vi "onTestExecution.vi"(7 "Name":string, 8 "error in (no error)":errorcluster, 11 "Test Runner in":refnum<class "Test Runner.lvclass">) -> (0 "error out":errorcluster, 3 "Test Runner out":refnum<class "Test Runner.lvclass">)   [LabVIEW 2013, in "Caraya.lvlib" / "Test Runner.lvclass"]
uses:
  Test Runner.lvclass
  Assert/Assert True.vi
  Assert/Assert.lvclass
  Test/Test.lvclass
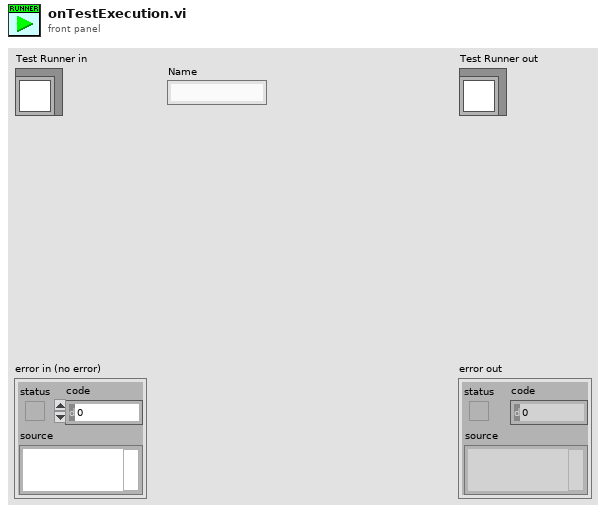
[diagram p1: front panel]
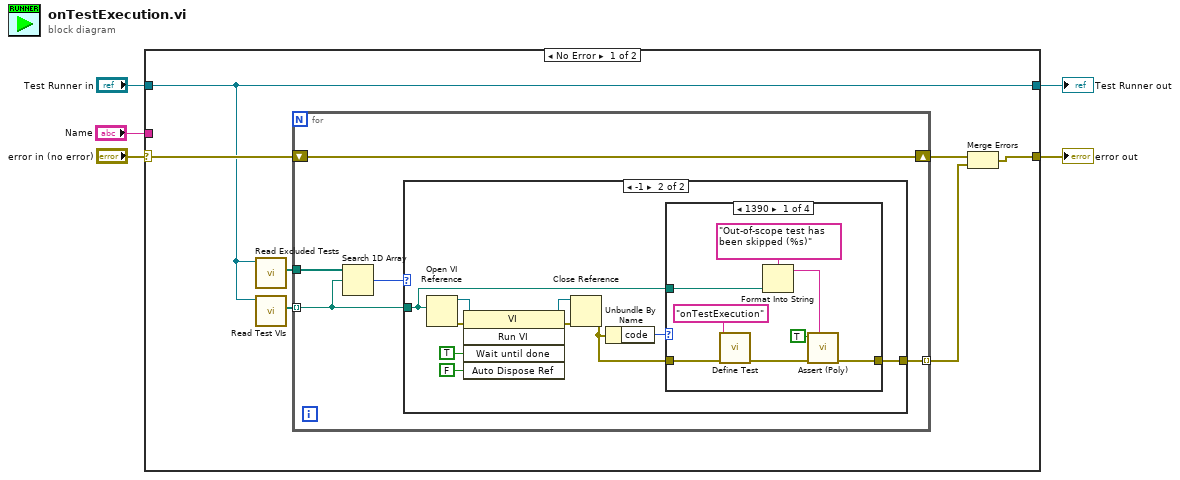
[diagram p0: block diagram]
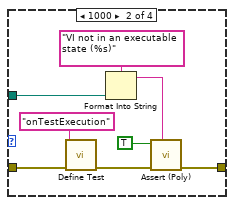
[diagram p3: hidden frame]
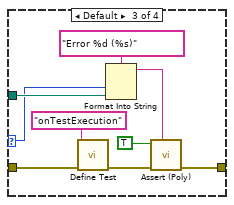
[diagram p4: hidden frame]
diagram:
  n1 = case shown="No Error" "error in (no error)" {
    selector: "error in (no error)" -> [w9 w55]
    tunnel: "Test Runner in" -> [w7 w54]
    tunnel: [w7 w54] -> w4
    tunnel: [w6 w55] -> w3
    tunnel: "Name" -> [_ _]
    frame No Error {
      n2 = call "Read Excluded Tests.vi"("Test Runner in"=w7) -> ("Excluded Tests"=w11:path[])  [unwired: 8 in, 2 out]
      n3 = call "Read Test VIs.vi"("Test Runner in"=w7) -> ("Test VIs"=w10:path[])  [unwired: 8 in, 2 out]
      n4 = for {
        tunnel: w10 -> [w16] mode=indexing
        tunnel: [w15] -> w12 mode=indexing
        tunnel: w11 -> [w17]
        shift-right: [w13] -> w8
        shift-left: w9 -> [w13]
        n5 = Search 1D Array(1D array=w17, element=w16) -> (index of element=w14:i32)  [unwired: 1 in]
        n6 = case shown="-1" w14 {
          tunnel: w16 -> [_ w19]
          tunnel: [_ w18] -> w15
          frame Default {
            # "Test is part of the exclusion list"
          }
          frame -1 {
            n7 = Open VI Reference(vi path=w19) -> (vi reference=w20:refnum<vi>, error out=w27:errorcluster)  [unwired: 5 in]
            n8 = invoke on="Invoke Node" class="VI" method="Run VI"(reference=w20, error in=w27, "Wait until done"=TRUE ("Wait Until Done"), "Auto Dispose Ref"=FALSE ("Auto Dispose Reference")) -> (reference out=w23:refnum<vi>, error out=w22:errorcluster)  [unwired: 1 in, 3 out]
            n9 = Close Reference(reference=w23, error in (no error)=w22) -> (error out=w21:errorcluster)
            n10 = Unbundle By Name(w21) -> ("code"=w24:i32)
            n11 = case shown="1390" w24 {
              selector: w24 -> [_ _ w47 _]
              tunnel: w21 -> [w30 w37 w44 w53]
              tunnel: [w34 w42 w51 w53] -> w18
              tunnel: w19 -> [w32 w40 w49 _]
              frame 1390 {
                n12 = call "Define Test.vi"("error in (no error)"=w30, "Label (VI Title)"="onTestExecution" ("Label")) -> ("error out"=w29:errorcluster)  [unwired: 9 in]
                n13 = Format Into String(format string="Out-of-scope test has been skipped (%s)" ("Label"), w32) -> (resulting string=w33:string)  [unwired: 2 in, 1 out]
                n14 = call-poly "Assert (Poly).vi"("Label"=w33, "error in (no error)"=w29, "True?"=TRUE) -> ("error out"=w34:errorcluster)  [unwired: 8 in]
              }
              frame 1000 {
                n15 = call "Define Test.vi"("error in (no error)"=w37, "Label (VI Title)"="onTestExecution" ("Label")) -> ("error out"=w36:errorcluster)  [unwired: 9 in]
                n16 = Format Into String(format string="VI not in an executable state (%s)" ("Label"), w40) -> (resulting string=w41:string)  [unwired: 2 in, 1 out]
                n17 = call-poly "Assert (Poly).vi"("Label"=w41, "error in (no error)"=w36, "True?"=TRUE) -> ("error out"=w42:errorcluster)  [unwired: 8 in]
              }
              frame Default {
                n18 = call "Define Test.vi"("error in (no error)"=w44, "Label (VI Title)"="onTestExecution" ("Label")) -> ("error out"=w45:errorcluster)  [unwired: 9 in]
                n19 = Format Into String(format string="Error %d (%s)" ("Label"), w47, w49) -> (resulting string=w50:string)  [unwired: 2 in, 1 out]
                n20 = call-poly "Assert (Poly).vi"("Label"=w50, "error in (no error)"=w45, "True?"=TRUE) -> ("error out"=w51:errorcluster)  [unwired: 8 in]
              }
              frame 0 {
              }
            }
          }
        }
      }
      n21 = Merge Errors(w8, w12) -> (w6:errorcluster)
    }
    frame Error {
    }
  }
  "error out" <- w3
  "Test Runner out" <- w4
